vi "ActiView806-Lores.vi"() -> ()   [LabVIEW 2020] (continued)
                  n599 = To Long Integer(number=w1270) -> (32bit integer=w1148:i32)
                  n600 = To Long Integer(number=w1305) -> (32bit integer=w1126:i32)
                  n601 = To Long Integer(number=w1306) -> (32bit integer=w1125:i32)
                  n602 = To Long Integer(number=w1304) -> (32bit integer=w1127:i32)
                  n603 = To Long Integer(number=w1290) -> (32bit integer=w1134:i32)
                  n604 = Multiply(x=w1292, y=100.0) -> (x*y=w1293:dbl)
                  n605 = To Long Integer(number=w1225) -> (32bit integer=w1216:i32)
                  n606 = Boolean To (0,1)(Boolean=w1267) -> (0, 1=w1268:i16)
                  n607 = To Long Integer(number=w1132) -> (32bit integer=w1130:i32)
                  n608 = To Long Integer(number=w1227) -> (32bit integer=w1214:i32)
                  n609 = To Long Integer(number=w1172) -> (32bit integer=w1213:i32)
                  n610 = Boolean To (0,1)(Boolean=w1266) -> (0, 1=w1265:i16)
                  n611 = To Long Integer(number=w1226) -> (32bit integer=w1215:i32)
                  n612 = To Long Integer(number=w1232) -> (32bit integer=w1224:i32)
                  n613 = To Long Integer(number=w1231) -> (32bit integer=w1223:i32)
                  n614 = Boolean To (0,1)(Boolean=w1229) -> (0, 1=w1219:i16)
                  n615 = To Long Integer(number=w1243) -> (32bit integer=w1120:i32)
                  n616 = To Long Integer(number=w1220) -> (32bit integer=w1221:i32)
                  n617 = To Long Integer(number=w1275) -> (32bit integer=w1259:i32)
                  n618 = Multiply(x=w1208, y=100.0) -> (x*y=w1207:dbl)
                  n619 = Boolean To (0,1)(Boolean=w1230) -> (0, 1=w1222:i16)
                  n620 = To Long Integer(number=w1299) -> (32bit integer=w1129:i32)
                  n621 = Multiply(x=w1262, y=100.0) -> (x*y=w1264:dbl)
                  n622 = To Long Integer(number=w1300) -> (32bit integer=w1128:i32)
                  n623 = To Long Integer(number=w1261) -> (32bit integer=w1138:i32)
                  n624 = Boolean To (0,1)(Boolean=w1228) -> (0, 1=w1217:i16)
                  n625 = To Long Integer(number=w1181) -> (32bit integer=w1179:i32)
                  n626 = To Long Integer(number=w1258) -> (32bit integer=w1212:i32)
                  n627 = To Long Integer(number=w1257) -> (32bit integer=w1178:i32)
                  n628 = To Long Integer(number=w1286) -> (32bit integer=w1122:i32)
                  n629 = To Long Integer(number=w1285) -> (32bit integer=w1123:i32)
                  n630 = To Long Integer(number=w1146) -> (32bit integer=w1144:i32)
                  n631 = To Long Integer(number=w1287) -> (32bit integer=w1260:i32)
                  n632 = To Long Integer(number=w1219) -> (32bit integer=w1210:i32)
                  n633 = To Long Integer(number=w1274) -> (32bit integer=w1177:i32)
                  n634 = To Long Integer(number=w1147) -> (32bit integer=w1142:i32)
                  n635 = To Long Integer(number=w1293) -> (32bit integer=w1133:i32)
                  n636 = To Long Integer(number=w1273) -> (32bit integer=w1176:i32)
                  n637 = To Long Integer(number=w1222) -> (32bit integer=w1211:i32)
                  n638 = To Long Integer(number=w1265) -> (32bit integer=w1151:i32)
                  n639 = To Long Integer(number=w1271) -> (32bit integer=w1175:i32)
                  n640 = To Long Integer(number=w1269) -> (32bit integer=w1150:i32)
                  n641 = To Long Integer(number=w1268) -> (32bit integer=w1149:i32)
                  n642 = Boolean To (0,1)(Boolean=w1244) -> (0, 1=w1245:i16)
                  n643 = To Long Integer(number=w1264) -> (32bit integer=w1152:i32)
                  n644 = To Long Integer(number=w1217) -> (32bit integer=w1209:i32)
                  n645 = To Long Integer(number=w1207) -> (32bit integer=w1218:i32)
                  n646 = To Long Integer(number=w1245) -> (32bit integer=w1153:i32)
                  n647 = Build Array(w1118, w1119, w1120, w1121, w1122, w1123, w1124, w1125, w1126, w1127, w1128, w1129, w1130, w1297, w1138, w1137, w1136, w1135, w1134, w1133, w1260, w1259, w1224, w1223, w1211, w1221, w1210, w1218, w1209, w1216, w1215, w1214, w1213, w1212, w1179, w1178, w1177, w1176, w1175, w1144, w1142, w1148, w1149, w1150, w1151, w1152, w1153, w1154) -> (w1233:i32[])
                  n648 = for {
                    shift-right: [w1421] -> w1238
                    shift-left: w1171 -> [w1423]
                    shift-right: [w1422] -> w1239
                    shift-left: w1164 -> [w1424]
                    tunnel: w1276 -> [w1420] mode=indexing
                    tunnel: w1165 -> [w1419]
                    tunnel: w1233 -> [w1417] mode=indexing
                    n649 = Number To Decimal String(number=w1417) -> (decimal integer string=w1418:string)  [unwired: 1 out]
                    n650 = call-poly <vilib>:"Write Key.vi"("section"=w1419, "error in (no error)"=w1423, "value"=w1418, "key"=w1420, "refnum"=w1424) -> ("error out"=w1421:errorcluster, "refnum out"=w1422:T19)  [unwired: 1 in, 4 out]
                  }
                  n651 = Array Size(array=w1187) -> (size(s)=w1193:i32)
                  n652 = Decrement(x=w1193) -> (x-1=w1189:i32)
                  n653 = for {
                    tunnel: w1240 -> [w1380] mode=indexing
                    shift-right: [w1383] -> w1235
                    shift-left: w1238 -> [w1384]
                    shift-right: [w1382] -> w1236
                    shift-left: w1239 -> [w1385]
                    tunnel: w1237 -> [w1381]
                    i -> [w1379]
                    n654 = case shown="9" w1379 {
                      tunnel: [w1386 w1387 w1388 w1389 w1390 w1392 w1393 w1395 w1396 w1397 w1398] -> w1378
                      frame 0, Default {
                        n655 = local read "MonFree"() -> (w1386:i32[])
                      }
                      frame 1 {
                        n656 = local read "RefFree"() -> (w1387:i32[])
                      }
                      frame 2 {
                        n657 = local read "BipFree"() -> (w1388:i32[])
                      }
                      frame 3 {
                        n658 = local read "AvgTrigSel"() -> (w1389:i32[])
                      }
                      frame 4 {
                        n659 = local read "MonFreeAvg1"() -> (w1391:i32)
                        n660 = Build Array(w1391) -> (w1390:i32[])
                      }
                      frame 5 {
                        n661 = local read "RefFreeAvg1"() -> (w1392:i32[])
                      }
                      frame 6 {
                        n662 = local read "MonFreeAvg2"() -> (w1394:i32)
                        n663 = Build Array(w1394) -> (w1393:i32[])
                      }
                      frame 7 {
                        n664 = local read "RefFreeAvg2"() -> (w1395:i32[])
                      }
                      frame 8 {
                        n665 = local read "AuxFree"() -> (w1396:i32[])
                      }
                      frame 9 {
                        n666 = local read "JazzFree"() -> (w1397:i32[])
                      }
                      frame 10 {
                        n667 = local read "AnaFree"() -> (w1398:i32[])
                      }
                    }
                    n668 = call "ArrayToCFG.vi"("Selector Array"=w1378) -> ("Cofiguration String"=w1377:string)
                    n669 = call-poly <vilib>:"Write Key.vi"("section"=w1381, "error in (no error)"=w1384, "value"=w1377, "key"=w1380, "refnum"=w1385) -> ("error out"=w1383:errorcluster, "refnum out"=w1382:T19)  [unwired: 1 in, 4 out]
                  }
                  n670 = for {
                    N: w1189 -> [_]
                    shift-right: [w1413] -> w1250
                    shift-left: w1236 -> [w1416]
                    shift-right: [w1414] -> w1249
                    shift-left: w1235 -> [w1415]
                    tunnel: w1234 -> [w1412]
                    tunnel: w1280 -> [w1411] mode=indexing
                    tunnel: w1187 -> [w1409] mode=indexing
                    n671 = Number To Decimal String(number=w1411) -> (decimal integer string=w1410:string)  [unwired: 1 out]
                    n672 = call-poly <vilib>:"Write Key.vi"("section"=w1412, "error in (no error)"=w1415, "value"=w1410, "key"=w1409, "refnum"=w1416) -> ("error out"=w1414:errorcluster, "refnum out"=w1413:T19)  [unwired: 1 in, 4 out]
                  }
                  n673 = local read "TCPaddAnas"() -> (w1186:bool)
                  n674 = Decrement(x=w1193) -> (x-1=w1192:i32)
                  n675 = local read "TCPaddSens"() -> (w1185:bool)
                  n676 = local read "TCPaddJazz"() -> (w1140:bool)
                  n677 = local read "TCPaddTrig"() -> (w1173:bool)
                  n678 = local read "TCPsubset"() -> (w1183:i8)
                  n679 = local read "TCPaddTP"() -> (w1184:bool)
                  n680 = local read "LocalPort"() -> (w1182:u16)
                  n681 = Path To String(path=w1248) -> (string=w1247:string)
                  n682 = Index Array(array=w1187, index=w1192) -> (element=w1188:string)
                  n683 = Boolean To (0,1)(Boolean=w1185) -> (0, 1=w1201:i16)
                  n684 = Boolean To (0,1)(Boolean=w1184) -> (0, 1=w1202:i16)
                  n685 = Boolean To (0,1)(Boolean=w1140) -> (0, 1=w1141:i16)
                  n686 = Boolean To (0,1)(Boolean=w1186) -> (0, 1=w1200:i16)
                  n687 = Boolean To (0,1)(Boolean=w1173) -> (0, 1=w1174:i16)
                  n688 = To Long Integer(number=w1183) -> (32bit integer=w1203:i32)
                  n689 = To Long Integer(number=w1182) -> (32bit integer=w1204:i32)
                  n690 = To Long Integer(number=w1202) -> (32bit integer=w1199:i32)
                  n691 = To Long Integer(number=w1201) -> (32bit integer=w1198:i32)
                  n692 = To Long Integer(number=w1141) -> (32bit integer=w1139:i32)
                  n693 = To Long Integer(number=w1200) -> (32bit integer=w1155:i32)
                  n694 = To Long Integer(number=w1174) -> (32bit integer=w1156:i32)
                  n695 = call-poly <vilib>:"Write Key.vi"("write raw string? (F)"=w1246, "section"=w1234, "error in (no error)"=w1249, "value"=w1247, "key"=w1188, "refnum"=w1250) -> ("error out"=w1196:errorcluster, "refnum out"=w1197:T19)  [unwired: 4 out]
                  n696 = Build Array(w1204, w1203, w1199, w1198, w1139, w1155, w1156) -> (w1205:i32[])
                  n697 = Wait (ms)(milliseconds to wait=u32 300) -> ()  [unwired: 1 out]
                  n698 = for {
                    shift-right: [w1373] -> w1195
                    shift-left: w1197 -> [w1376]
                    shift-right: [w1374] -> w1194
                    shift-left: w1196 -> [w1375]
                    tunnel: w1191 -> [w1372]
                    tunnel: w1205 -> [w1371] mode=indexing
                    tunnel: w1190 -> [w1369] mode=indexing
                    n699 = Number To Decimal String(number=w1371) -> (decimal integer string=w1370:string)  [unwired: 1 out]
                    n700 = call-poly <vilib>:"Write Key.vi"("section"=w1372, "error in (no error)"=w1375, "value"=w1370, "key"=w1369, "refnum"=w1376) -> ("error out"=w1374:errorcluster, "refnum out"=w1373:T19)  [unwired: 1 in, 4 out]
                  }
                  n701 = call <vilib>:"Close Config Data.vi"("error in (no error)"=w1194, "write file if changed (T)"=w1284, "refnum"=w1195) -> ("error out"=w1278:errorcluster)  [unwired: 8 out]
                  n702 = call <vilib>:"General Error Handler.vi"("type of dialog (OK msg:1)"=w1254, "error in (no error)"=w1278) -> ("error out"=w1279:errorcluster)  [unwired: 1 in, 12 out]
                  n703 = Unbundle By Name(w1279) -> ("status"=w1277:bool)
                  n704 = case shown="False" w1277 {
                    tunnel: w1117 -> [w1407 _]
                    frame False {
                      n705 = Path To String(path=w1407) -> (string=w1408:string)
                      n706 = local write "Current Filepath"(w1408) -> ()
                    }
                    frame True {
                    }
                  }
                  "Write CFG" <- w1284
                }
                frame True {
                }
              }
            }
          }
          n707 = local read "Charts/Graphs"() -> (w427:T2)
          n708 = Index Array(array=w344, index #1=2 ("index"), index #2=5 ("index")) -> (element #1=w273:i8, element #2=w276:i8)
          n709 = Index Array(array=w378, index #1=6 ("index")) -> (element #1=w376:i32, element #2=w375:i32)  [unwired: 1 in]
          n710 = local read "Reference"() -> (w421:i8)
          n711 = local read "Channels"() -> (w419:i8)
          n712 = call "AVTCP-Save FGV.vi"() -> ("Value out"=w249:bool)  [unwired: 7 in]
          n713 = call "AVTCP-Start FGV.vi"() -> ("Value out"=w250:bool)  [unwired: 7 in]
          n714 = To Unsigned Word Integer(number=w276) -> (unsigned 16bit integer=w339:u16)
          n715 = property class="VI"("Front Panel Window:Closeable"=TRUE) -> ()  [unwired: 2 in, 2 out]
          n716 = Or(x="Start Saving", y=w249) -> (x .or. y?=w247:bool)
          n717 = case shown="0, Default" w273 {
            tunnel: [i8 3 ("x") i8 4 ("x")] -> w272
            frame 0, Default {
            }
            frame 1 {
            }
          }
          n718 = case shown="\"About ActiView\", Default" w427 {
            tunnel: [T1."Monopolar" ("Left Sidebar") T1."Bipolar" ("Left Sidebar") T1."Offset" ("Left Sidebar") T1."Average" ("Left Sidebar") T1."Sensors" ("Left Sidebar") T1."Jazz" ("Left Sidebar") T1."Analog" ("Left Sidebar") T1."Initialization" ("Left Sidebar")] -> w303
            frame "Monopolar Display" {
            }
            frame "Bipolar Leads" {
            }
            frame "Electrode Offset" {
            }
            frame "Event Related Average" {
            }
            frame "Auxiliary Sensors" {
            }
            frame "Jazz Eyetracker" {
            }
            frame "Analog Input Box" {
            }
            frame "About ActiView", Default {
            }
          }
          n719 = Format Into String(format string=w381, w376) -> (resulting string=w379:string)  [unwired: 2 in, 1 out]
          n720 = Format Into String(format string=w381, w375) -> (resulting string=w383:string)  [unwired: 2 in, 1 out]
          n721 = local read "OffsetScale"() -> (w417:i8)
          n722 = call-poly <vilib>:"Set Cursor.vi"("icon"=w339) -> ("error out"=w341:errorcluster)  [unwired: 2 in, 8 out]
          n723 = local write "Mon Filter Reset"(w392) -> ()
          n724 = local write "Bip Filter Reset"(w392) -> ()
          n725 = local write "Write CFG"(w392) -> ()
          n726 = local write "Stop"(w392) -> ()
          n727 = Equal?(x=w419, y=i8 14 ("x")) -> (x = y?=w423:bool)
          n728 = Compound Arithmetic op=OR("Edit", "Start", w250, w247) -> (w248:bool)
          n729 = Equal?(x=w421, y=i8 8) -> (x = y?=w422:bool)
          n730 = local write "Start Saving"(w247) -> ()
          n731 = Equal?(x=w272, y=w417) -> (x = y?=w418:bool)
          n732 = Path To String(path=w372) -> (string=w371:string)
          n733 = Select(t=w252, s=w422, f=w253) -> (s? t:f=w426:T5)
          n734 = Concatenate Strings(w379, " / " ("Substring"), w383) -> (→"Pause Off/On":string)
          n735 = Select(t=w252, s=w423, f=w253) -> (s? t:f=w425:T5)
          n736 = property on="Pause Saving" class="Bool (strict)"("Disabled"=w253) -> ()  [unwired: 2 in, 2 out]
          n737 = local write "Full Range"(w418) -> ()
          n738 = local write "Filepath"(w371) -> ()
          n739 = local write "Left Sidebar"(w303) -> ()
          n740 = property on="RefFree" class="LstBox (strict)"("Disabled"=w426) -> ()  [unwired: 2 in, 2 out]
          n741 = property on="MonFree" class="LstBox (strict)"("Disabled"=w425) -> ()  [unwired: 2 in, 2 out]
          n742 = call <vilib>:"General Error Handler.vi"("type of dialog (OK msg:1)"=w340, "error in (no error)"=w341) -> ()  [unwired: 1 in, 13 out]
          n743 = Wait (ms)(milliseconds to wait=u32 200 ("millisecond timer value")) -> ()  [unwired: 1 out]
        }
        n744 = Index Array(array=w203) -> (element #1=w208:i8, element #2=w168:i8, element #3=w207:i8, element #4=w205:i8, element #5=w193:i8, element #6=w192:i8, element #7=w166:i8, element #8=w165:i8)  [unwired: 8 in]
        n745 = Index Array(array=w204) -> (element #1=w223:i32, element #2=w235:i32, element #3=w234:i32, element #4=w220:i32, element #5=w171:i32, element #6=w173:i32, element #7=w190:i32, element #8=w174:i32)  [unwired: 8 in]
        n746 = To Unsigned Byte Integer(number=w193) -> (unsigned 8bit integer=w195:u8)
        n747 = To Unsigned Word Integer(number=w192) -> (unsigned 16bit integer=w194:u16)
        n748 = Bundle By Name(cluster=w211, "Warning"=w208, "Motherboard"=w168, "ElecGain"=w207, "RespSwitch"=w205, "LineWidth"=w195, "Cursor"=w194, "PopupKiller"=w166, "BreathBelt"=w165) -> (w210:T6)
        n749 = In Range and Coerce(upper limit=15, x=w173, lower limit=1) -> (coerced(x)=w188:i32)  [unwired: 1 out]
        n750 = Not Equal To 0?(x=w171) -> (x != 0?=w170:bool)
        n751 = Not Equal To 0?(x=w220) -> (x != 0?=w219:bool)
        n752 = To Unsigned Long Integer(number=w188) -> (unsigned 32bit integer=w172:u32)
        n753 = To Byte Integer(number=w223) -> (8bit integer=w209:i8)
        n754 = Not Equal To 0?(x=w234) -> (x != 0?=w233:bool)
        n755 = Not Equal To 0?(x=w235) -> (x != 0?=w232:bool)
        n756 = Bundle By Name(cluster=w186, "Save Subset"=w209, "Add Touchproofs"=w232, "Add Sensors"=w233, "Add Jazz"=w219, "Add Anas"=w170, "Save Box"=w172, "PauseOff"=w190, "PauseOn"=w174, "Save Path"=w175) -> (w236:T7)
      }
      frame 1 {
        w1509 = 0.2035  # 5th order sinc
        w1475 = i8 0 items=["All 256 Chan ", "A + B", "C + D", "E + F", "G + H"] ("Offset")
        w1638 = i8 0 items=["None (raw)", "Avg of 256", "Avg 1-224", "Avg 1-160", "Avg 1-128", "Avg 1-64", "Avg 1-32", "Avg of Displ", "Free Choice"] ("Reference")
        w1501 = 0 ("f")
        w1504 = 4  # Jazz Chan
        w1654 = FALSE  # Config Changed
        w1665 = FALSE  # Stop Running
        w1670 = 2  # Go to State 2 Initialize
        # "Jazz ?"
        # "Multibox?"
        # "Anabox?"
        # "Config Changed"
        # "Sensors?"
        n757 = flat-sequence {
          tunnel: w1454 -> [w2147]
          tunnel: [w2147] -> w1453
          tunnel: [w2164] -> w1612
          tunnel: [w2163] -> w1566
          tunnel: [w2162] -> w1564
          tunnel: [w2161] -> w1563
          tunnel: [w2159] -> w1524
          tunnel: [w2158] -> w1523
          tunnel: [w2157] -> w1508
          tunnel: "JazzOn" -> [w2153]
          tunnel: w1453 -> [w2149]
          tunnel: w1612 -> [w2210]
          tunnel: [w2217] -> w1565
          tunnel: w1566 -> [w2217]
          tunnel: w1564 -> [w2216]
          tunnel: w1563 -> [w2215]
          tunnel: [w2215] -> w1457
          tunnel: w1524 -> [w2214]
          tunnel: [w2214] -> w1469
          tunnel: w1523 -> [w2213]
          tunnel: w1508 -> [w2212]
          tunnel: [w2212] -> w1461
          frame #0 {
            n758 = global write "StopJazzIni.glb" "JazzIniStop"(FALSE) -> ()
          }
          frame #1 {
            w2155 = i64 1900544  # Max Samples in 2 sec
            w2160 = i64 0  # Integer 64
            n759 = call "Act_Open.vi"("Buffer Size in Byte"=w2149, "JazzOn"=w2153) -> ("Handle Out"=w2150:i64, "Buffer Size in Words"=w2151:i64, "RingBuffer"=w2152:i32[])
            n760 = Select(t=w2155, s=w2153, f=i64 256 ("Display Blocksize In")) -> (s? t:f=w2154:i64)
            n761 = while {
              tunnel: w2152 -> [w2191]
              tunnel: [w2190] -> w2163
              tunnel: w2151 -> [w2189]
              shift-right: [w2188] -> _
              shift-left: w2160 -> [w2182]
              tunnel: w2160 -> [w2187]
              tunnel: [w2173] -> w2164
              tunnel: [w2181] -> w2162
              tunnel: [w2180] -> w2161
              tunnel: [w2178] -> w2159
              tunnel: [w2177] -> w2158
              tunnel: [w2176] -> w2157
              tunnel: w2154 -> [w2175]
              tunnel: w2150 -> [w2172]
              i -> [w2184]
              stop <- w2174 stop-if-true
              n762 = Equal To 0?(x=w2184) -> (x = 0?=w2183:bool)
              n763 = call "Act_Pointer.vi"("First Iteration"=w2183, "Handle In"=w2172, "Display Blocksize In"=w2175, "Buffer Size"=w2189, "Old Total Displayed"=w2187, "Old Total Buffered"=w2182) -> ("Data Ready"=w2185:bool, "No Incoming Data"=w2179:bool, "New Total Buffered"=w2188:i64, "Handle Out"=w2173:i64)  [unwired: 1 out]
              n764 = case shown="True" w2185 {
                tunnel: w2191 -> [_ w2204]
                tunnel: [i8 -1 ("t") w2203] -> w2190
                tunnel: [FALSE TRUE] -> w2186
                tunnel: [w2193 w2206] -> w2181
                tunnel: [w2192 w2198] -> w2180
                tunnel: [w2192 w2200] -> w2178
                tunnel: [w2193 w2199] -> w2177
                tunnel: [w2192 w2197] -> w2176
                frame False {
                  w2192 = TRUE
                  w2193 = "?" ("f")
                  n765 = Wait (ms)(milliseconds to wait=u32 10) -> ()  [unwired: 1 out]
                }
                frame True {
                  n766 = call "Act_Mode.vi"("Serial Data"=w2204) -> ("SpeedMode"=w2203:i8, "Mk2 ?"=w2198:bool, "GSR16Hz ?"=w2200:bool, "Jazz ?"=w2197:bool)
                  n767 = property on="Battery" class="Slide (strict)"("Visible"=w2198) -> ()  [unwired: 2 in, 2 out]
                  n768 = Not(x=w2198) -> (.not. x?=w2205:bool)
                  n769 = property on="Low Battery" class="Bool (strict)"("Visible"=w2205) -> ()  [unwired: 2 in, 2 out]
                  n770 = Select(t="nanoS", s=w2200, f="Ohm") -> (s? t:f=w2199:string)
                  n771 = Select(t="Mk2", s=w2198, f="Mk1") -> (s? t:f=w2206:string)
                }
              }
              n772 = Or(x=w2179, y=w2186) -> (x .or. y?=w2174:bool)
              n773 = global write "StopJazzIni.glb" "JazzIniStop"(w2174) -> ()
            }
            n774 = case shown="True" w2153 {
              frame False {
              }
              frame True {
                n775 = while {
                  shift-left: TRUE ("NoRefWarning") -> [w2167]
                  shift-right: [w2166] -> _
                  stop <- w2166 stop-if-true
                  n776 = Wait (ms)(milliseconds to wait=u32 10) -> ()  [unwired: 1 out]
                  n777 = case shown="True" w2167 {
                    tunnel: [w2169 w2171] -> w2166
                    frame False {
                      n778 = global read "StopJazzIni.glb" "JazzIniStop"() -> (w2169:bool)
                    }
                    frame True {
                      n779 = call "JazzIni.vi"() -> ("Ready"=w2170:bool)  [unwired: 1 out]
                      n780 = Not(x=w2170) -> (.not. x?=w2171:bool)
                    }
                  }
                }
              }
            }
          }
          frame #2 {
            # "JazzRec ?"
            # "GSR16Hz ?"
            # "Version Mk?"
            n781 = global write "StopJazzIni.glb" "JazzIniStop"(FALSE) -> ()
            n782 = call "Act_Close.vi"("Handle In"=w2210) -> ()
            "Speed Mode" <- w2217
            "AD-box" <- w2216
            "GSR units" <- w2213
          }
        }
        n783 = local read "Decimation"() -> (w1511:i8)
        n784 = local read "TCPsubset"() -> (w1580:i8)
        n785 = local read "Reference"() -> (w1623:i8)
        n786 = local read "Channels"() -> (w1624:i8)
        n787 = local read "MonFree"() -> (w1621:i32[])
        n788 = local read "JazzFree"() -> (w1480:i32[])
        n789 = local read "AuxFree"() -> (w1542:i32[])
        n790 = local read "AnaFree"() -> (w1543:i32[])
        n791 = local read "RefFree"() -> (w1620:i32[])
        n792 = local read "BipFree"() -> (w1569:i32[])
        n793 = local read "Offset"() -> (w1622:i8)
        n794 = case shown="True" w1457 {
          tunnel: [w1710 w1894] -> w1579
          tunnel: [w1711 w1893] -> w1576
          tunnel: [w1709 w1892] -> w1578
          tunnel: [w1708 w1891] -> w1577
          tunnel: [w1704 w1890] -> w1506
          tunnel: [w1703 w1889] -> w1570
          tunnel: [w1705 w1888] -> w1463
          tunnel: [w1700 w1887] -> w1477
          tunnel: [w1699 w1886] -> w1494
          tunnel: [w1702 w1885] -> w1572
          tunnel: [w1701 w1884] -> w1571
          tunnel: w1565 -> [w1706 w1883]
          tunnel: [w1707 w1882] -> w1443
          tunnel: [w1698 w1880] -> w1573
          tunnel: [w1697 w1881] -> w1575
          tunnel: w1459 -> [w1696 w1879]
          tunnel: [w1695 w1879] -> w1458
          frame False {
            # "Old Mk1 version"
            n795 = case shown="9" w1706 {
              selector: w1706 -> [w1715 w1731 w1746 w1761 w1776 w1791 w1806 w1821 w1836 w1852 w1867]
              tunnel: [232 ("Mon Channels") 256 ("Mon Channels") 128 ("Mon Channels") 64 ("Mon Channels") 32 ("Mon Channels") 232 ("Mon Channels") 104 ("Mon Channels") 40 ("Mon Channels") 8 ("Mon Channels") 232 ("Mon Channels") 232 ("Mon Channels")] -> w1702
              tunnel: [8 ("Bip Channels") 0 ("Bip Channels") 0 ("Bip Channels") 0 ("Bip Channels") 0 ("Bip Channels") 8 ("Bip Channels") 8 ("Bip Channels") 8 ("Bip Channels") 8 ("Bip Channels") 8 ("Bip Channels") 8 ("Bip Channels")] -> w1701
              tunnel: [8 ("Aux Channels") 0 ("Aux Channels") 0 ("Aux Channels") 0 ("Aux Channels") 0 ("Aux Channels") 8 ("Aux Channels") 8 ("Aux Channels") 8 ("Aux Channels") 8 ("Aux Channels") 8 ("Aux Channels") 8 ("Aux Channels")] -> w1700
              tunnel: [w1726 w1730 w1745 w1760 w1775 w1790 w1805 w1820 w1835 w1851 w1878] -> w1711
              tunnel: [i32[] [] ("Disabled Items []") i32[] [0, 13] ("Disabled Items []") i32[] [0, 1, 2, 9, 10, 11, 12, 13] ("Disabled Items []") i32[] [0, 1, 2, 3, 7, 8, 9, 10, 11, 12, 13] ("Disabled Items []") i32[] [0, 1, 2, 3, 4, 6, 7, 8, 9, 10, 11, 12, 13] ("Disabled Items []") i32[] [0, 1, 12] ("Disabled Items []") i32[] [0, 1, 2, 3, 8, 9, 10, 11, 12] ("Disabled Items []") i32[] [0, 1, 2, 3, 4, 6, 7, 8, 9, 10, 11, 12] ("Disabled Items []") i32[] [0, 1, 2, 3, 4, 5, 6, 7, 8, 9, 10, 11, 12] ("Disabled Items []") i32[] [0, 1, 12] ("Disabled Items []") i32[] [] ("Disabled Items []")] -> w1710
              tunnel: [i32[] [] ("Disabled Items []") i32[] [1] ("Disabled Items []") i32[] [1, 2, 3] ("Disabled Items []") i32[] [1, 2, 3, 4] ("Disabled Items []") i32[] [1, 2, 3, 4, 5] ("Disabled Items []") i32[] [1, 2] ("Disabled Items []") i32[] [1, 2, 3, 4] ("Disabled Items []") i32[] [1, 2, 3, 4, 5] ("Disabled Items []") i32[] [1, 2, 3, 4, 5, 6] ("Disabled Items []") i32[] [1] ("Disabled Items []") i32[] [] ("Disabled Items []")] -> w1709
              tunnel: [i32[] [] ("Disabled Items []") i32[] [] ("Disabled Items []") i32[] [3, 4] ("Disabled Items []") i32[] [2, 3, 4] ("Disabled Items []") i32[] [2, 3, 4] ("Disabled Items []") i32[] [] ("Disabled Items []") i32[] [3, 4] ("Disabled Items []") i32[] [2, 3, 4] ("Disabled Items []") i32[] [2, 3, 4] ("Disabled Items []") i32[] [] ("Disabled Items []") i32[] [] ("Disabled Items []")] -> w1708
              tunnel: [32 ("Aux Channels") 0 ("Aux Channels") 0 ("Aux Channels") 0 ("Aux Channels") 0 ("Aux Channels") 0 ("Aux Channels") 0 ("Aux Channels") 0 ("Aux Channels") 0 ("Aux Channels") 32 ("Aux Channels") 32 ("Aux Channels")] -> w1699
              tunnel: [0 ("ADC Rate") 2048 ("ADC Rate") 4096 ("ADC Rate") 8192 ("ADC Rate") 16384 ("ADC Rate") 2048 ("ADC Rate") 4096 ("ADC Rate") 8192 ("ADC Rate") 16384 ("ADC Rate") 2048 ("ADC Rate") 0 ("ADC Rate")] -> w1705
              tunnel: [0 ("Nr of Chan") 258 ("Nr of Chan") 130 ("Nr of Chan") 66 ("Nr of Chan") 34 ("Nr of Chan") 258 ("Nr of Chan") 130 ("Nr of Chan") 66 ("Nr of Chan") 34 ("Nr of Chan") 290 ("Nr of Chan") 0 ("Nr of Chan")] -> w1704
              tunnel: [0 ("Nr of Chan") 2 ("Nr of Chan") 4 ("Nr of Chan") 8 ("Nr of Chan") 16 ("Nr of Chan") 2 ("Nr of Chan") 4 ("Nr of Chan") 8 ("Nr of Chan") 16 ("Nr of Chan") 2 ("Nr of Chan") 0 ("Nr of Chan")] -> w1703
              tunnel: [w1715 w1731 w1746 w1761 w1776 w1791 w1806 w1821 w1836 w1852 w1867] -> w1707
              tunnel: [i32[] [] ("Disabled Items []") i32[] [] ("Disabled Items []") i32[] [0, 1] ("Disabled Items []") i32[] [0, 1, 2] ("Disabled Items []") i32[] [0, 1, 2, 3] ("Disabled Items []") i32[] [0] ("Disabled Items []") i32[] [0, 1, 2] ("Disabled Items []") i32[] [0, 1, 2, 3] ("Disabled Items []") i32[] [0, 1, 2, 3, 4, 5] ("Disabled Items []") i32[] [0] ("Disabled Items []") i32[] [] ("Disabled Items []")] -> w1698
              tunnel: [w1713 w1729 w1744 w1759 w1774 w1789 w1803 w1819 w1834 w1850 w1865] -> w1697
              tunnel: w1696 -> [w1712 w1727 w1742 w1757 w1772 w1787 w1802 w1817 w1832 w1847 w1863]
              tunnel: [w1712 w1727 w1742 w1757 w1772 w1787 w1802 w1817 w1832 w1847 w1864] -> w1695
              frame -1, Default {
                w1713 = i8 0 items=["A1 - H32 (256)", "A1 - E32 (160)", "A1 - D32 (128)", "A1 - B32 (64)", "A1 - A32 (32)", "A1 - A16 (16)", "A1 -A8 (8)", "None (0) "] ("TCP subset:")
                w1726 = i8 0 items=["All 256 Chan ", "A-G (224)", "A-E (160)", "ABCD (128)", "A+B (64)", "A (32)", "B (32)", "C (32)", "D (32)", "E (32)", "F (32)", "G (32)", "H(32)", "EXG (8)", "Free Choice"] ("Channels")
              }
              frame 0 {
                w1729 = i8 0 items=["A1 - H32 (256)", "A1 - E32 (160)", "A1 - D32 (128)", "A1 - B32 (64)", "A1 - A32 (32)", "A1 - A16 (16)", "A1 -A8 (8)", "None (0) "] ("TCP subset:")
                w1730 = i8 1 items=["All 264 Chan ", "A-H (256)", "A-E (160)", "ABCD (128)", "A+B (64)", "A (32)", "B (32)", "C (32)", "D (32)", "E (32)", "F (32)", "G (32)", "H(32)", "EXG (8)", "Free Choice"] ("Channels")
              }
              frame 1 {
                w1744 = i8 2 items=["A1 - H32 (256)", "A1 - E32 (160)", "A1 - D32 (128)", "A1 - B32 (64)", "A1 - A32 (32)", "A1 - A16 (16)", "A1 -A8 (8)", "None (0) "] ("TCP subset:")
                w1745 = i8 3 items=["All 264 Chan ", "A-H (256)", "A-E (160)", "ABCD (128)", "A+B (64)", "A (32)", "B (32)", "C (32)", "D (32)", "E (32)", "F (32)", "G (32)", "H(32)", "EXG (8)", "Free Choice"] ("Channels")
              }
              frame 2 {
                w1759 = i8 3 items=["A1 - H32 (256)", "A1 - E32 (160)", "A1 - D32 (128)", "A1 - B32 (64)", "A1 - A32 (32)", "A1 - A16 (16)", "A1 -A8 (8)", "None (0) "] ("TCP subset:")
                w1760 = i8 4 items=["All 264 Chan ", "A-H (256)", "A-E (160)", "ABCD (128)", "A+B (64)", "A (32)", "B (32)", "C (32)", "D (32)", "E (32)", "F (32)", "G (32)", "H(32)", "EXG (8)", "Free Choice"] ("Channels")
              }
              frame 3 {
                w1774 = i8 4 items=["A1 - H32 (256)", "A1 - E32 (160)", "A1 - D32 (128)", "A1 - B32 (64)", "A1 - A32 (32)", "A1 - A16 (16)", "A1 -A8 (8)", "None (0) "] ("TCP subset:")
                w1775 = i8 5 items=["All 264 Chan ", "A-H (256)", "A-E (160)", "ABCD (128)", "A+B (64)", "A (32)", "B (32)", "C (32)", "D (32)", "E (32)", "F (32)", "G (32)", "H(32)", "EXG (8)", "Free Choice"] ("Channels")
              }
              frame 4 {
                w1789 = i8 1 items=["A1 - H32 (256)", "A1 - E32 (160)", "A1 - D32 (128)", "A1 - B32 (64)", "A1 - A32 (32)", "A1 - A16 (16)", "A1 -A8 (8)", "None (0) "] ("TCP subset:")
                w1790 = i8 2 items=["All 264 Chan ", "A-H (256)", "A-E (160)", "ABCD (128)", "A+B (64)", "A (32)", "B (32)", "C (32)", "D (32)", "E (32)", "F (32)", "G (32)", "H(32)", "EXG (8)", "Free Choice"] ("Channels")
              }
              frame 5 {
                w1803 = i8 3 items=["A1 - H32 (256)", "A1 - E32 (160)", "A1 - D32 (128)", "A1 - B32 (64)", "A1 - A32 (32)", "A1 - A16 (16)", "A1 -A8 (8)", "None (0) "] ("TCP subset:")
                w1805 = i8 4 items=["All 264 Chan ", "A-H (256)", "A-E (160)", "ABCD (128)", "A+B (64)", "A (32)", "B (32)", "C (32)", "D (32)", "E (32)", "F (32)", "G (32)", "H(32)", "EXG (8)", "Free Choice"] ("Channels")
              }
              frame 6 {
                w1819 = i8 4 items=["A1 - H32 (256)", "A1 - E32 (160)", "A1 - D32 (128)", "A1 - B32 (64)", "A1 - A32 (32)", "A1 - A16 (16)", "A1 -A8 (8)", "None (0) "] ("TCP subset:")
                w1820 = i8 5 items=["All 264 Chan ", "A-H (256)", "A-E (160)", "ABCD (128)", "A+B (64)", "A (32)", "B (32)", "C (32)", "D (32)", "E (32)", "F (32)", "G (32)", "H(32)", "EXG (8)", "Free Choice"] ("Channels")
              }
              frame 7 {
                w1834 = i8 6 items=["A1 - H32 (256)", "A1 - E32 (160)", "A1 - D32 (128)", "A1 - B32 (64)", "A1 - A32 (32)", "A1 - A16 (16)", "A1 -A8 (8)", "None (0) "] ("TCP subset:")
                w1835 = i8 14 items=["All 264 Chan ", "A-H (256)", "A-E (160)", "ABCD (128)", "A+B (64)", "A (32)", "B (32)", "C (32)", "D (32)", "E (32)", "F (32)", "G (32)", "H(32)", "EXG (8)", "Free Choice"] ("Channels")
              }
              frame 8 {
                w1850 = i8 1 items=["A1 - H32 (256)", "A1 - E32 (160)", "A1 - D32 (128)", "A1 - B32 (64)", "A1 - A32 (32)", "A1 - A16 (16)", "A1 -A8 (8)", "None (0) "] ("TCP subset:")
                w1851 = i8 2 items=["All 264 Chan ", "A-H (256)", "A-E (160)", "ABCD (128)", "A+B (64)", "A (32)", "B (32)", "C (32)", "D (32)", "E (32)", "F (32)", "G (32)", "H(32)", "EXG (8)", "Free Choice"] ("Channels")
              }
              frame 9 {
                w1862 = u32 3  # Error Code In
                w1865 = i8 0 items=["A1 - H32 (256)", "A1 - E32 (160)", "A1 - D32 (128)", "A1 - B32 (64)", "A1 - A32 (32)", "A1 - A16 (16)", "A1 -A8 (8)", "None (0) "] ("TCP subset:")
                w1878 = i8 0 items=["All 256 Chan ", "A-G (224)", "A-E (160)", "ABCD (128)", "A+B (64)", "A (32)", "B (32)", "C (32)", "D (32)", "E (32)", "F (32)", "G (32)", "H(32)", "EXG (8)", "Free Choice"] ("Channels")
                n796 = call "Act_Error_Jazz.vi"("Error Code In"=w1862, "error in (no error)"=w1863) -> ("error out"=w1864:errorcluster)  [unwired: 2 out]
              }
            }
          }
          frame True {
            # "New Mk2 version"
            n797 = case shown="15" w1883 {
              selector: w1883 -> [w1898 w1912 w1926 w1940 w1954 w1968 w1982 w1997 w2011 w2024 w2038 w2052 w2066 w2080 w2095 w2108 w2122]
              tunnel: [256 ("Mon Channels") 128 ("Mon Channels") 128 ("Mon Channels") 128 ("Mon Channels") 128 ("Mon Channels") 256 ("Mon Channels") 128 ("Mon Channels") 64 ("Mon Channels") 32 ("Mon Channels") 256 ("Mon Channels") 128 ("Mon Channels") 256 ("Mon Channels") 128 ("Mon Channels") 256 ("Mon Channels") 128 ("Mon Channels") 256 ("Mon Channels") 256 ("Mon Channels")] -> w1885
              tunnel: [8 ("Bip Channels") 8 ("Bip Channels") 8 ("Bip Channels") 8 ("Bip Channels") 8 ("Bip Channels") 8 ("Bip Channels") 8 ("Bip Channels") 8 ("Bip Channels") 8 ("Bip Channels") 8 ("Bip Channels") 8 ("Bip Channels") 8 ("Bip Channels") 8 ("Bip Channels") 8 ("Bip Channels") 8 ("Bip Channels") 8 ("Bip Channels") 8 ("Bip Channels")] -> w1884
              tunnel: [8 ("Aux Channels") 8 ("Aux Channels") 8 ("Aux Channels") 8 ("Aux Channels") 8 ("Aux Channels") 8 ("Aux Channels") 8 ("Aux Channels") 8 ("Aux Channels") 8 ("Aux Channels") 8 ("Aux Channels") 8 ("Aux Channels") 8 ("Aux Channels") 8 ("Aux Channels") 8 ("Aux Channels") 8 ("Aux Channels") 8 ("Aux Channels") 8 ("Aux Channels")] -> w1887
              tunnel: [w1897 w1911 w1925 w1939 w1953 w1967 w1981 w1996 w2010 w2023 w2037 w2051 w2065 w2079 w2094 w2107 w2121] -> w1893
              tunnel: [i32[] [] ("Disabled Items []") i32[] [0, 1, 2, 9, 10, 11, 12] ("Disabled Items []") i32[] [0, 1, 2, 9, 10, 11, 12] ("Disabled Items []") i32[] [0, 1, 2, 9, 10, 11, 12] ("Disabled Items []") i32[] [0, 1, 2, 9, 10, 11, 12] ("Disabled Items []") i32[] [] ("Disabled Items []") i32[] [0, 1, 2, 9, 10, 11, 12] ("Disabled Items []") i32[] [0, 1, 2, 3, 7, 8, 9, 10, 11, 12] ("Disabled Items []") i32[] [0, 1, 2, 3, 4, 6, 7, 8, 9, 10, 11, 12] ("Disabled Items []") i32[] [] ("Disabled Items []") i32[] [0, 1, 2, 9, 10, 11, 12] ("Disabled Items []") i32[] [] ("Disabled Items []") i32[] [0, 1, 2, 9, 10, 11, 12] ("Disabled Items []") i32[] [] ("Disabled Items []") i32[] [0, 1, 2, 9, 10, 11, 12] ("Disabled Items []") i32[] [] ("Disabled Items []") i32[] [] ("Disabled Items []")] -> w1894
              tunnel: [i32[] [] ("Disabled Items []") i32[] [1, 2, 3] ("Disabled Items []") i32[] [1, 2, 3] ("Disabled Items []") i32[] [1, 2, 3] ("Disabled Items []") i32[] [1, 2, 3] ("Disabled Items []") i32[] [] ("Disabled Items []") i32[] [1, 2, 3] ("Disabled Items []") i32[] [1, 2, 3, 4] ("Disabled Items []") i32[] [1, 2, 3, 4, 5] ("Disabled Items []") i32[] [] ("Disabled Items []") i32[] [1, 2, 3] ("Disabled Items []") i32[] [] ("Disabled Items []") i32[] [1, 2, 3] ("Disabled Items []") i32[] [] ("Disabled Items []") i32[] [1, 2, 3] ("Disabled Items []") i32[] [] ("Disabled Items []") i32[] [] ("Disabled Items []")] -> w1892
              tunnel: [i32[] [] ("Disabled Items []") i32[] [3, 4] ("Disabled Items []") i32[] [3, 4] ("Disabled Items []") i32[] [3, 4] ("Disabled Items []") i32[] [3, 4] ("Disabled Items []") i32[] [] ("Disabled Items []") i32[] [3, 4] ("Disabled Items []") i32[] [2, 3, 4] ("Disabled Items []") i32[] [2, 3, 4] ("Disabled Items []") i32[] [] ("Disabled Items []") i32[] [3, 4] ("Disabled Items []") i32[] [] ("Disabled Items []") i32[] [3, 4] ("Disabled Items []") i32[] [] ("Disabled Items []") i32[] [3, 4] ("Disabled Items []") i32[] [] ("Disabled Items []") i32[] [] ("Disabled Items []")] -> w1891
              tunnel: [32 ("Aux Channels") 0 ("Aux Channels") 0 ("Aux Channels") 0 ("Aux Channels") 0 ("Aux Channels") 0 ("Aux Channels") 0 ("Aux Channels") 0 ("Aux Channels") 0 ("Aux Channels") 32 ("Aux Channels") 0 ("Aux Channels") 0 ("Aux Channels") 0 ("Aux Channels") 0 ("Aux Channels") 0 ("Aux Channels") 0 ("Aux Channels") 0 ("Aux Channels")] -> w1886
              tunnel: [0 ("ADC Rate") 2048 ("ADC Rate") 2048 ("ADC Rate") 2048 ("ADC Rate") 2048 ("ADC Rate") 2048 ("ADC Rate") 4096 ("ADC Rate") 8192 ("ADC Rate") 16384 ("ADC Rate") 2048 ("ADC Rate") 8192 ("ADC Rate") 4096 ("ADC Rate") 8192 ("ADC Rate") 8192 ("ADC Rate") 16384 ("ADC Rate") 2048 ("ADC Rate") 2048 ("ADC Rate")] -> w1888
              tunnel: [0 ("Nr of Chan") 610 ("Nr of Chan") 610 ("Nr of Chan") 610 ("Nr of Chan") 610 ("Nr of Chan") 282 ("Nr of Chan") 154 ("Nr of Chan") 90 ("Nr of Chan") 58 ("Nr of Chan") 314 ("Nr of Chan") 154 ("Nr of Chan") 282 ("Nr of Chan") 154 ("Nr of Chan") 282 ("Nr of Chan") 154 ("Nr of Chan") 562 ("Nr of Chan") 562 ("Nr of Chan")] -> w1890
              tunnel: [0 ("Nr of Chan") 2 ("Nr of Chan") 2 ("Nr of Chan") 2 ("Nr of Chan") 2 ("Nr of Chan") 2 ("Nr of Chan") 4 ("Nr of Chan") 8 ("Nr of Chan") 16 ("Nr of Chan") 2 ("Nr of Chan") 8 ("Nr of Chan") 4 ("Nr of Chan") 8 ("Nr of Chan") 8 ("Nr of Chan") 16 ("Nr of Chan") 2 ("Nr of Chan") 2 ("Nr of Chan")] -> w1889
              tunnel: [w1898 w1912 w1926 w1940 w1954 w1968 w1982 w1997 w2011 w2024 w2038 w2052 w2066 w2080 w2095 w2108 w2122] -> w1882
              tunnel: [w1896 w1910 w1924 w1938 w1952 w1966 w1980 w1993 w2008 w2022 w2036 w2050 w2064 w2078 w2093 w2106 w2120] -> w1881
              tunnel: [i32[] [] ("Disabled Items []") i32[] [0, 1] ("Disabled Items []") i32[] [0, 1] ("Disabled Items []") i32[] [0, 1] ("Disabled Items []") i32[] [0, 1] ("Disabled Items []") i32[] [] ("Disabled Items []") i32[] [0, 1] ("Disabled Items []") i32[] [0, 1, 2] ("Disabled Items []") i32[] [0, 1, 2, 3] ("Disabled Items []") i32[] [] ("Disabled Items []") i32[] [0, 1] ("Disabled Items []") i32[] [] ("Disabled Items []") i32[] [0, 1] ("Disabled Items []") i32[] [] ("Disabled Items []") i32[] [0, 1] ("Disabled Items []") i32[] [] ("Disabled Items []") i32[] [] ("Disabled Items []")] -> w1880
              frame -1, Default {
                w1896 = i8 0 items=["A1 - H32 (256)", "A1 - E32 (160)", "A1 - D32 (128)", "A1 - B32 (64)", "A1 - A32 (32)", "A1 - A16 (16)", "A1 -A8 (8)", "None (0) "] ("TCP subset:")
                w1897 = i8 0 items=["All 264 Chan ", "A-H (256)", "A-E (160)", "ABCD (128)", "A+B (64)", "A (32)", "B (32)", "C (32)", "D (32)", "E (32)", "F (32)", "G (32)", "H(32)", "EXG (8)", "Free Choice"] ("Channels")
              }
              frame 0 {
                w1910 = i8 2 items=["A1 - H32 (256)", "A1 - E32 (160)", "A1 - D32 (128)", "A1 - B32 (64)", "A1 - A32 (32)", "A1 - A16 (16)", "A1 -A8 (8)", "None (0) "] ("TCP subset:")
                w1911 = i8 3 items=["All 264 Chan ", "A-H (256)", "A-E (160)", "ABCD (128)", "A+B (64)", "A (32)", "B (32)", "C (32)", "D (32)", "E (32)", "F (32)", "G (32)", "H(32)", "EXG (8)", "Free Choice"] ("Channels")
              }
              frame 1 {
                w1924 = i8 2 items=["A1 - H32 (256)", "A1 - E32 (160)", "A1 - D32 (128)", "A1 - B32 (64)", "A1 - A32 (32)", "A1 - A16 (16)", "A1 -A8 (8)", "None (0) "] ("TCP subset:")
                w1925 = i8 3 items=["All 264 Chan ", "A-H (256)", "A-E (160)", "ABCD (128)", "A+B (64)", "A (32)", "B (32)", "C (32)", "D (32)", "E (32)", "F (32)", "G (32)", "H(32)", "EXG (8)", "Free Choice"] ("Channels")
              }
              frame 2 {
                w1938 = i8 2 items=["A1 - H32 (256)", "A1 - E32 (160)", "A1 - D32 (128)", "A1 - B32 (64)", "A1 - A32 (32)", "A1 - A16 (16)", "A1 -A8 (8)", "None (0) "] ("TCP subset:")
                w1939 = i8 3 items=["All 264 Chan ", "A-H (256)", "A-E (160)", "ABCD (128)", "A+B (64)", "A (32)", "B (32)", "C (32)", "D (32)", "E (32)", "F (32)", "G (32)", "H(32)", "EXG (8)", "Free Choice"] ("Channels")
              }
              frame 3 {
                w1952 = i8 2 items=["A1 - H32 (256)", "A1 - E32 (160)", "A1 - D32 (128)", "A1 - B32 (64)", "A1 - A32 (32)", "A1 - A16 (16)", "A1 -A8 (8)", "None (0) "] ("TCP subset:")
                w1953 = i8 3 items=["All 264 Chan ", "A-H (256)", "A-E (160)", "ABCD (128)", "A+B (64)", "A (32)", "B (32)", "C (32)", "D (32)", "E (32)", "F (32)", "G (32)", "H(32)", "EXG (8)", "Free Choice"] ("Channels")
              }
              frame 4 {
                w1966 = i8 0 items=["A1 - H32 (256)", "A1 - E32 (160)", "A1 - D32 (128)", "A1 - B32 (64)", "A1 - A32 (32)", "A1 - A16 (16)", "A1 -A8 (8)", "None (0) "] ("TCP subset:")
                w1967 = i8 1 items=["All 264 Chan ", "A-H (256)", "A-E (160)", "ABCD (128)", "A+B (64)", "A (32)", "B (32)", "C (32)", "D (32)", "E (32)", "F (32)", "G (32)", "H(32)", "EXG (8)", "Free Choice"] ("Channels")
              }
              frame 5 {
                w1980 = i8 2 items=["A1 - H32 (256)", "A1 - E32 (160)", "A1 - D32 (128)", "A1 - B32 (64)", "A1 - A32 (32)", "A1 - A16 (16)", "A1 -A8 (8)", "None (0) "] ("TCP subset:")
                w1981 = i8 3 items=["All 264 Chan ", "A-H (256)", "A-E (160)", "ABCD (128)", "A+B (64)", "A (32)", "B (32)", "C (32)", "D (32)", "E (32)", "F (32)", "G (32)", "H(32)", "EXG (8)", "Free Choice"] ("Channels")
              }
              frame 6 {
                w1993 = i8 3 items=["A1 - H32 (256)", "A1 - E32 (160)", "A1 - D32 (128)", "A1 - B32 (64)", "A1 - A32 (32)", "A1 - A16 (16)", "A1 -A8 (8)", "None (0) "] ("TCP subset:")
                w1996 = i8 4 items=["All 264 Chan ", "A-H (256)", "A-E (160)", "ABCD (128)", "A+B (64)", "A (32)", "B (32)", "C (32)", "D (32)", "E (32)", "F (32)", "G (32)", "H(32)", "EXG (8)", "Free Choice"] ("Channels")
              }
              frame 7 {
                w2008 = i8 4 items=["A1 - H32 (256)", "A1 - E32 (160)", "A1 - D32 (128)", "A1 - B32 (64)", "A1 - A32 (32)", "A1 - A16 (16)", "A1 -A8 (8)", "None (0) "] ("TCP subset:")
                w2010 = i8 5 items=["All 264 Chan ", "A-H (256)", "A-E (160)", "ABCD (128)", "A+B (64)", "A (32)", "B (32)", "C (32)", "D (32)", "E (32)", "F (32)", "G (32)", "H(32)", "EXG (8)", "Free Choice"] ("Channels")
              }
              frame 8 {
                w2022 = i8 0 items=["A1 - H32 (256)", "A1 - E32 (160)", "A1 - D32 (128)", "A1 - B32 (64)", "A1 - A32 (32)", "A1 - A16 (16)", "A1 -A8 (8)", "None (0) "] ("TCP subset:")
                w2023 = i8 1 items=["All 264 Chan ", "A-H (256)", "A-E (160)", "ABCD (128)", "A+B (64)", "A (32)", "B (32)", "C (32)", "D (32)", "E (32)", "F (32)", "G (32)", "H(32)", "EXG (8)", "Free Choice"] ("Channels")
              }
              frame 9 {
                w2036 = i8 2 items=["A1 - H32 (256)", "A1 - E32 (160)", "A1 - D32 (128)", "A1 - B32 (64)", "A1 - A32 (32)", "A1 - A16 (16)", "A1 -A8 (8)", "None (0) "] ("TCP subset:")
                w2037 = i8 3 items=["All 264 Chan ", "A-H (256)", "A-E (160)", "ABCD (128)", "A+B (64)", "A (32)", "B (32)", "C (32)", "D (32)", "E (32)", "F (32)", "G (32)", "H(32)", "EXG (8)", "Free Choice"] ("Channels")
              }
              frame 10 {
                w2050 = i8 0 items=["A1 - H32 (256)", "A1 - E32 (160)", "A1 - D32 (128)", "A1 - B32 (64)", "A1 - A32 (32)", "A1 - A16 (16)", "A1 -A8 (8)", "None (0) "] ("TCP subset:")
                w2051 = i8 1 items=["All 264 Chan ", "A-H (256)", "A-E (160)", "ABCD (128)", "A+B (64)", "A (32)", "B (32)", "C (32)", "D (32)", "E (32)", "F (32)", "G (32)", "H(32)", "EXG (8)", "Free Choice"] ("Channels")
              }
              frame 11 {
                w2064 = i8 2 items=["A1 - H32 (256)", "A1 - E32 (160)", "A1 - D32 (128)", "A1 - B32 (64)", "A1 - A32 (32)", "A1 - A16 (16)", "A1 -A8 (8)", "None (0) "] ("TCP subset:")
                w2065 = i8 3 items=["All 264 Chan ", "A-H (256)", "A-E (160)", "ABCD (128)", "A+B (64)", "A (32)", "B (32)", "C (32)", "D (32)", "E (32)", "F (32)", "G (32)", "H(32)", "EXG (8)", "Free Choice"] ("Channels")
              }
              frame 12 {
                w2078 = i8 0 items=["A1 - H32 (256)", "A1 - E32 (160)", "A1 - D32 (128)", "A1 - B32 (64)", "A1 - A32 (32)", "A1 - A16 (16)", "A1 -A8 (8)", "None (0) "] ("TCP subset:")
                w2079 = i8 1 items=["All 264 Chan ", "A-H (256)", "A-E (160)", "ABCD (128)", "A+B (64)", "A (32)", "B (32)", "C (32)", "D (32)", "E (32)", "F (32)", "G (32)", "H(32)", "EXG (8)", "Free Choice"] ("Channels")
              }
              frame 13 {
                w2093 = i8 2 items=["A1 - H32 (256)", "A1 - E32 (160)", "A1 - D32 (128)", "A1 - B32 (64)", "A1 - A32 (32)", "A1 - A16 (16)", "A1 -A8 (8)", "None (0) "] ("TCP subset:")
                w2094 = i8 3 items=["All 264 Chan ", "A-H (256)", "A-E (160)", "ABCD (128)", "A+B (64)", "A (32)", "B (32)", "C (32)", "D (32)", "E (32)", "F (32)", "G (32)", "H(32)", "EXG (8)", "Free Choice"] ("Channels")
              }
              frame 14 {
                w2106 = i8 0 items=["A1 - H32 (256)", "A1 - E32 (160)", "A1 - D32 (128)", "A1 - B32 (64)", "A1 - A32 (32)", "A1 - A16 (16)", "A1 -A8 (8)", "None (0) "] ("TCP subset:")
                w2107 = i8 1 items=["All 264 Chan ", "A-H (256)", "A-E (160)", "ABCD (128)", "A+B (64)", "A (32)", "B (32)", "C (32)", "D (32)", "E (32)", "F (32)", "G (32)", "H(32)", "EXG (8)", "Free Choice"] ("Channels")
              }
              frame 15 {
                w2120 = i8 0 items=["A1 - H32 (256)", "A1 - E32 (160)", "A1 - D32 (128)", "A1 - B32 (64)", "A1 - A32 (32)", "A1 - A16 (16)", "A1 -A8 (8)", "None (0) "] ("TCP subset:")
                w2121 = i8 1 items=["All 264 Chan ", "A-H (256)", "A-E (160)", "ABCD (128)", "A+B (64)", "A (32)", "B (32)", "C (32)", "D (32)", "E (32)", "F (32)", "G (32)", "H(32)", "EXG (8)", "Free Choice"] ("Channels")
              }
            }
          }
        }
        n798 = In Range and Coerce(upper limit=i8 13 ("y"), x=w1443, lower limit=i8 4 ("y")) -> (In Range?=w1446:bool)  [unwired: 1 out]
        n799 = Compound Arithmetic op=AND(w1446, w1461, "JazzOn") -> (w1445:bool)
        n800 = Select(t=w1504, s=w1445, f=w1501) -> (s? t:f=w1505:i32)
        n801 = Select(t=9 ("Nr of Chan"), s=w1445, f=w1501) -> (s? t:f=w1493:i32)
        n802 = To Byte Integer(number=w1573) -> (8bit integer=w1583:i8[])
        n803 = Add(x=w1506, y=w1505) -> (x+y=w1507:i32)
        n804 = To Byte Integer(number=w1577) -> (8bit integer=w1642:i8[])
        n805 = Search 1D Array(1D array=w1583, element=w1580) -> (index of element=w1582:i32)  [unwired: 1 out]
        n806 = To Byte Integer(number=w1578) -> (8bit integer=w1646:i8[])
        n807 = Search 1D Array(1D array=w1642, element=w1622) -> (index of element=w1641:i32)  [unwired: 1 out]
        n808 = Less Than 0?(x=w1582) -> (x < 0?=w1581:bool)
        n809 = Less Than 0?(x=w1641) -> (x < 0?=w1640:bool)
        n810 = Search 1D Array(1D array=w1646, element=w1623) -> (index of element=w1645:i32)  [unwired: 1 out]
        n811 = To Byte Integer(number=w1579) -> (8bit integer=w1650:i8[])
        n812 = Add(x=w1571, y=w1572) -> (x+y=w1464:i32)
        n813 = Select(t=w1580, s=w1581, f=w1575) -> (s? t:f=w1574:i8)
        n814 = Select(t=w1622, s=w1640, f=w1475) -> (s? t:f=w1639:i8)
        n815 = Less Than 0?(x=w1645) -> (x < 0?=w1644:bool)
        n816 = Scale By Power Of 2(n=w1511, x=1) -> (x*2^n=w1609:i32)
        n817 = Search 1D Array(1D array=w1650, element=w1624) -> (index of element=w1649:i32)  [unwired: 1 out]
        n818 = Select(t=w1623, s=w1644, f=w1638) -> (s? t:f=w1643:i8)
        n819 = Less Than 0?(x=w1649) -> (x < 0?=w1648:bool)
        n820 = local read "Charts/Graphs"() -> (w1468:T2)
        n821 = Unbundle By Name(w1503) -> ("Speed Mode"=w1562:i8)
        n822 = Equal?(x=w1443, y=i8 8) -> (x = y?=w1618:bool)
        n823 = Less Than 0?(x=w1443) -> (x < 0?=w1456:bool)
        n824 = Quotient & Remainder(x=w1463, y=2048) -> (floor(x/y)=w1521:i32)  [unwired: 1 out]
        n825 = Quotient & Remainder(x=w1463, y=w1609) -> (floor(x/y)=w1610:i32)  [unwired: 1 out]
        n826 = Select(t=w1624, s=w1648, f=w1576) -> (s? t:f=w1647:i8)
        n827 = Decrement(x=w1521) -> (x-1=w1520:i32)
        n828 = To Byte Integer(number=w1520) -> (8bit integer=w1519:i8)
        n829 = Not(x=w1445) -> (.not. x?=w1466:bool)
        n830 = Not(x=w1456) -> (.not. x?=w1495:bool)
        n831 = Equal?(x=w1468, y=T2."Jazz Eyetracker" ("Charts/Graphs")) -> (x = y?=w1467:bool)
        n832 = Or(x=w1618, y=w1456) -> (x .or. y?=w1496:bool)
        n833 = Not Equal?(x=w1562, y=w1443) -> (x != y?=w1652:bool)
        n834 = To Double Precision Float(number=w1610) -> (double precision float=w1436:dbl)
        n835 = Less Or Equal To 0?(x=w1463) -> (x <= 0?=w1516:bool)
        n836 = Subtract(x=w1511, y=w1519) -> (x-y=w1518:i8)
        n837 = And(x=w1467, y=w1466) -> (x .and. y?=w1465:bool)
        n838 = Not(x=w1446) -> (.not. x?=w1540:bool)
        n839 = Compound Arithmetic op=OR(w1446, w1456, w1457) -> (w1474:bool)
        n840 = Decrement(x=w1518) -> (x-1=w1476:i8)
        n841 = Multiply(x=w1509, y=w1436) -> (x*y=w1611:dbl)
        n842 = call "AVTCP-Sample Rate FGV.vi"("Value in"=w1436) -> ()  [unwired: 6 in, 1 out]
        n843 = local read "ScreenLength"() -> (w1514:i32)
        n844 = Compound Arithmetic op=OR(w1655, w1652, w1465) -> (w1625:bool)
        n845 = Compound Arithmetic op=AND(w1540, w1495, w1457) -> (w1439:bool)
        n846 = for {
          N: w1464 -> [_]
          tunnel: [w2221] -> w1584 mode=indexing
          i -> [w2221]
        }
        n847 = Less Or Equal To 0?(x=w1476) -> (x <= 0?=w1517:bool)
        n848 = local write "Bandwidth (3dB)"(w1611) -> ()
        n849 = local write "Sample Rate"(w1436) -> ()
        n850 = Bundle By Name(cluster=w1503, "Mark2"=w1457, "GSR16Hz"=w1469, "JazzRec"=w1461, "Speed Mode"=w1443, "ADC Rate"=w1463, "ADC Channels"=w1507, "Screen Ratio"=w1570, "Decimate Ratio"=w1609, "Mon Channels"=w1572, "Bip Channels"=w1571, "Aux Channels"=w1477, "Jazz Channels"=w1493, "Ana Channels"=w1494) -> (w1442:T7)
        n851 = Or(x=w1517, y=w1516) -> (x .or. y?=w1515:bool)
        n852 = case shown="False" w1515 {
          tunnel: [w1688 i32[] [] ("Disabled Items []")] -> w1512
          tunnel: [w1689 w1693] -> w1513
          tunnel: w1514 -> [w1690 w1693]
          tunnel: w1476 -> [w1687 _]
          frame False {
            n853 = To Long Integer(number=w1687) -> (32bit integer=w1686:i32)
            n854 = Greater?(x=w1686, y=w1690) -> (0:w1691:bool)
            n855 = for {
              N: w1686 -> [_]
              tunnel: [w1692] -> w1688 mode=indexing
              i -> [w1692]
            }
            n856 = Select(t=w1686, s=w1691, f=w1690) -> (s? t:f=w1689:i32)
          }
          frame True {
          }
        }
        n857 = for {
          tunnel: w1584 -> [w2259]
          shift-right: [w2255] -> w1614
          shift-left: i32[] [] -> [w2257]
          tunnel: w1621 -> [w2253] mode=indexing
          n858 = Search 1D Array(1D array=w2259, element=w2253) -> (index of element=w2258:i32)  [unwired: 1 out]
          n859 = Greater Or Equal To 0?(x=w2258) -> (x >= 0?=w2256:bool)
          n860 = Build Array (concatenate)(w2257, w2253) -> (w2254:i32[])
          n861 = Select(t=w2254, s=w2256, f=w2257) -> (s? t:f=w2255:i32[])
        }
        n862 = for {
          tunnel: w1584 -> [w2228]
          shift-right: [w2224] -> w1636
          shift-left: i32[] [] -> [w2226]
          tunnel: w1620 -> [w2222] mode=indexing
          n863 = Search 1D Array(1D array=w2228, element=w2222) -> (index of element=w2227:i32)  [unwired: 1 out]
          n864 = Greater Or Equal To 0?(x=w2227) -> (x >= 0?=w2225:bool)
          n865 = Build Array (concatenate)(w2226, w2222) -> (w2223:i32[])
          n866 = Select(t=w2223, s=w2225, f=w2226) -> (s? t:f=w2224:i32[])
        }
        n867 = property on="ScreenLength" class="Ring (strict)"("Disabled Items []"=w1512) -> ()  [unwired: 2 in, 2 out]
        n868 = local write "ScreenLength"(w1513) -> ()
        n869 = Or(x=w1445, y=w1456) -> (x .or. y?=w1470:bool)
        n870 = Array Size(array=w1614) -> (size(s)=w1617:i32)
        n871 = case shown="False" w1456 {
          tunnel: w1445 -> [w1685 _]
          frame False {
            n872 = local write "JazzOn"(w1685) -> ()
          }
          frame True {
          }
        }
        n873 = Equal To 0?(x=w1617) -> (x = 0?=w1616:bool)
        n874 = Select(t=i32[] [0], s=w1616, f=w1614) -> (s? t:f=w1613:i32[])
        n875 = local read "RefFreeAvg1"() -> (w1608:i32[])
        n876 = case shown="0, Default" w1443 {
